vi "subVI_PhenotypeParalysis.vi"(6 "Start frame #":i32=50, 8 "Nb of frame to analyze":i32=580, 9 "Threshold Phenotype WT vs Paralyzed":dbl=120000.0 format="%#_13g", 10 "Threshold to binarize worm":i32, 11 "Path":path=path "C:/Users/aguillaume3/Desktop/TEST/Videos/20190614GA Serotonin paralysis on chip/N2/21 38 15 1 .avi") -> (2 "Mutant?":i32, 3 "Sum of diff":i32)   [LabVIEW 2019]
uses:
  <vilib>/vision/NI_Vision_Development_Module.lvlib
panel:
  out "Result":string
  out "Histogram":T1(graph)
  out "Image 4":T2(plugin-control)
  out "Frame #":i32
  out "Nb of frames":i32
  out "Image 3":T2(plugin-control)
  out "Image 2":T2(plugin-control)
  # "Inputs"
  # "Outputs"
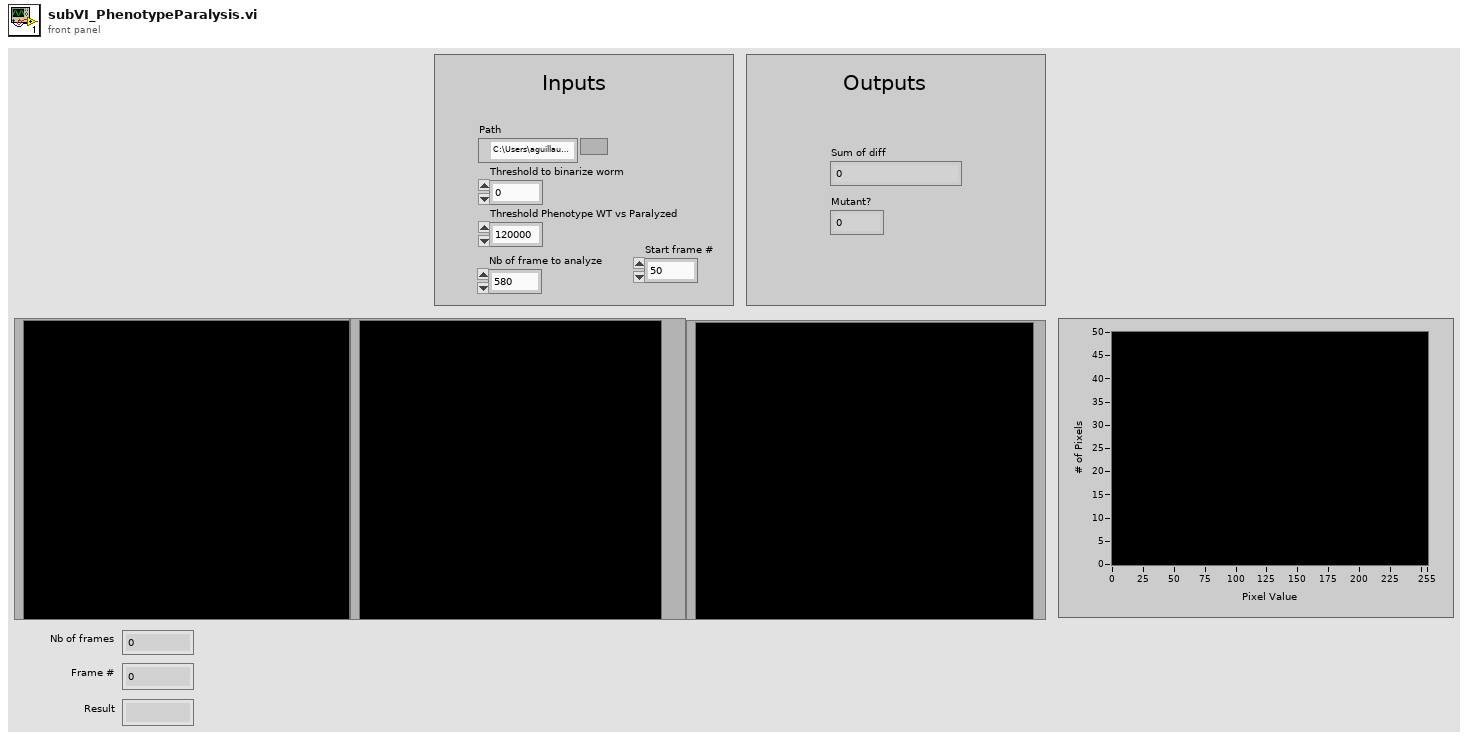
[diagram p1: front panel]
types:
  T1 = cluster{"Starting Value":sgl, "Incremental Value":sgl, "Histogram":u32[]}
  T2 = typedef "IMAQ Image.ctl" = refnum<image>
  T3 = typedef "Image Type" = u32
  T4 = typedef "IMAQ AVI2 Refnum.ctl" = refnum<k20>
  T5 = cluster{"Mean Value":sgl, "Standard Variation":sgl, "Minimal Value":sgl, "Maximal Value":sgl, "Area (calibrated)":sgl, "Area (pixels)":u32, "%":sgl, "Calibration Valid":bool}
  T6 = cluster{"histogram":u32[], "Minimal Value":sgl, "Maximal Value":sgl, "Starting Value":sgl, "Interval Width":sgl, "Mean Value":sgl, "Standard  Variation":sgl, "Area (pixels)":i32}
  T7 = cluster{"histogram[0]":u32, "histogram[1]":u32, "histogram[2]":u32, "histogram[3]":u32, "histogram[4]":u32, "histogram[5]":u32, "histogram[6]":u32, "histogram[7]":u32, "histogram[8]":u32}
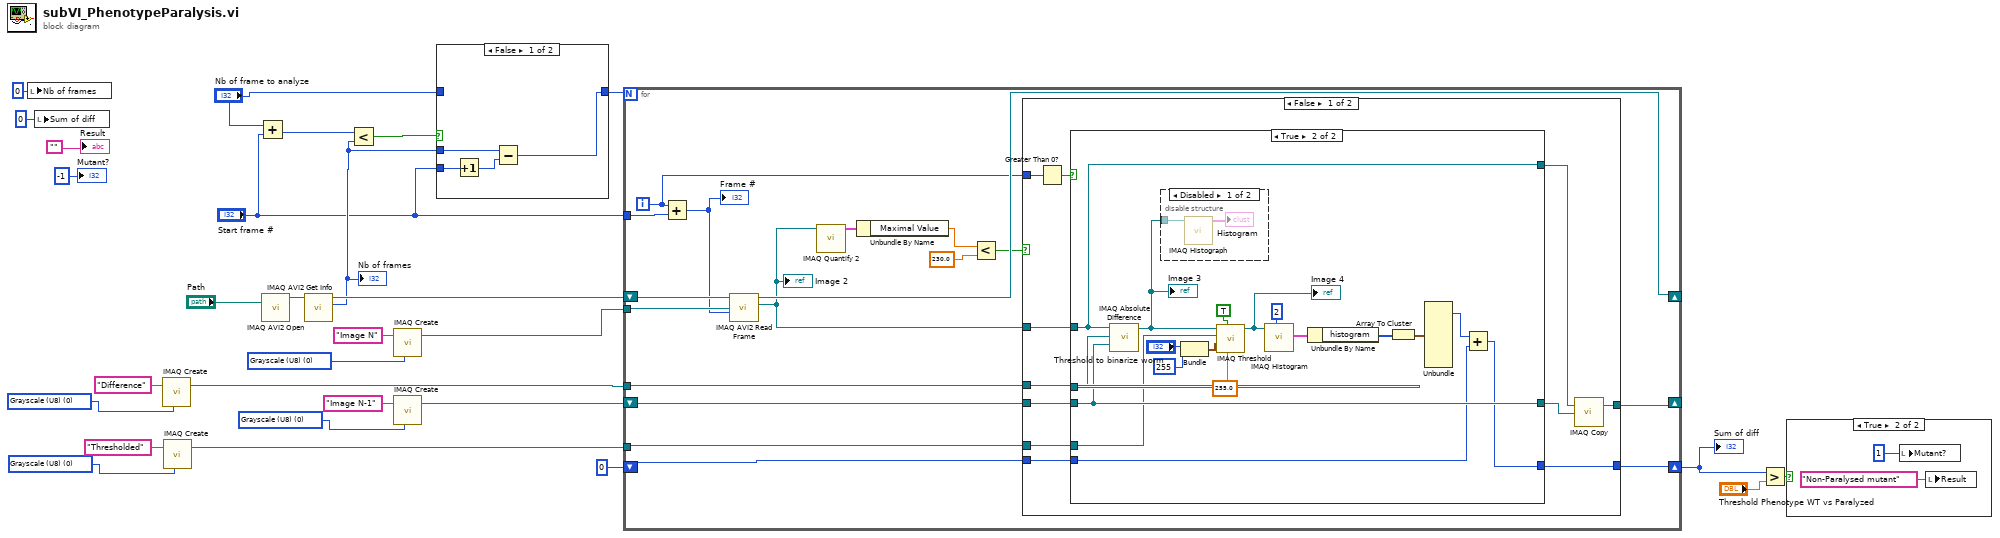
[diagram p0: block diagram]
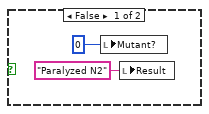
[diagram p3: hidden frame]
diagram:
  w18 = T3 0 items=["Grayscale (U8)", "Grayscale (I16)", "Grayscale (SGL)", "Complex (CSG)", "RGB (U32)", "HSL (U32)", "RGB (U64)", "Grayscale (U16)"] ("Image Type")
  w22 = T3 0 items=["Grayscale (U8)", "Grayscale (I16)", "Grayscale (SGL)", "Complex (CSG)", "RGB (U32)", "HSL (U32)", "RGB (U64)", "Grayscale (U16)"] ("Image Type")
  w25 = T3 0 items=["Grayscale (U8)", "Grayscale (I16)", "Grayscale (SGL)", "Complex (CSG)", "RGB (U32)", "HSL (U32)", "RGB (U64)", "Grayscale (U16)"] ("Image Type")
  w28 = T3 0 items=["Grayscale (U8)", "Grayscale (I16)", "Grayscale (SGL)", "Complex (CSG)", "RGB (U32)", "HSL (U32)", "RGB (U64)", "Grayscale (U16)"] ("Image Type")
  n1 = local write "Nb of frames"(0 ("Sum of diff")) -> ()
  n2 = local write "Sum of diff"(0 ("Sum of diff")) -> ()
  n3 = call "IMAQ Create"("Image Name"="Difference", "Image Type"=w22) -> ("New Image"=w21:T2)  [unwired: 3 in, 1 out]
  n4 = call "IMAQ Create"("Image Name"="Thresholded", "Image Type"=w18) -> ("New Image"=w17:T2)  [unwired: 3 in, 1 out]
  n5 = Add(x="Nb of frame to analyze", y="Start frame #") -> (x+y=w6:i32)
  n6 = call "IMAQ AVI2 Open"("AVI File Path"="Path") -> ("AVI Refnum"=w13:T4)  [unwired: 9 in, 1 out]
  n7 = call "IMAQ AVI2 Get Info"("AVI Refnum"=w13) -> ("Number of Frames"=w2:u32, "AVI Refnum (duplicate)"=w12:T4)  [unwired: 6 in, 3 out]
  "Nb of frames" <- w2
  n8 = Less?(x=w6, y=w2) -> (x < y?=w5:bool)
  n9 = call "IMAQ Create"("Image Name"="Image N", "Image Type"=w28) -> ("New Image"=w27:T2)  [unwired: 3 in, 1 out]
  n10 = call "IMAQ Create"("Image Name"="Image N-1", "Image Type"=w25) -> ("New Image"=w24:T2)  [unwired: 3 in, 1 out]
  n11 = case shown="False" w5 {
    tunnel: "Nb of frame to analyze" -> [_ w34]
    tunnel: [w32 w34] -> w3
    tunnel: w2 -> [w33 _]
    tunnel: "Start frame #" -> [w31 _]
    frame False {
      n12 = Increment(x=w31) -> (x+1=w30:i32)
      n13 = Subtract(x=w33, y=w30) -> (x-y=w32:u32)
    }
    frame True {
    }
  }
  n14 = for {
    N: w3 -> [_]
    shift-right: [w51] -> _
    shift-left: w12 -> [w50]
    tunnel: w27 -> [w49]
    shift-right: [w47] -> _
    shift-left: w24 -> [w48]
    tunnel: w21 -> [w46]
    shift-right: [w44] -> w10
    shift-left: 0 ("Numeric") -> [w45]
    tunnel: w17 -> [w42]
    tunnel: "Start frame #" -> [w40]
    i -> [w41]
    n15 = Add(x=w41, y=w40) -> (x+y=w43:i32)
    "Frame #" <- w43
    n16 = call "IMAQ AVI2 Read Frame"("Frame Number"=w43, "Image"=w49, "AVI Refnum"=w50) -> ("Image Out"=w38:T2, "AVI Refnum (duplicate)"=w51:T4)  [unwired: 6 in, 1 out]
    "Image 2" <- w38
    n17 = call "IMAQ Quantify 2"("Image"=w38) -> ("Global Report"=w39:T5)  [unwired: 8 in, 2 out]
    n18 = Unbundle By Name(w39) -> ("Maximal Value"=w37:sgl)
    n19 = Less?(x=w37, y=sgl 230.0) -> (x < y?=w35:bool)
    n20 = case shown="False" w35 {
      tunnel: w48 -> [w62 w87]
      tunnel: [w61 w87] -> w47
      tunnel: w46 -> [w60 _]
      tunnel: w45 -> [w59 w86]
      tunnel: [w58 w86] -> w44
      tunnel: w42 -> [w57 _]
      tunnel: w38 -> [w53 _]
      tunnel: w41 -> [w52 _]
      frame False {
        n21 = Greater Than 0?(x=w52) -> (x > 0?=w54:bool)
        n22 = case shown="True" w54 {
          tunnel: w62 -> [w64 w81]
          tunnel: w53 -> [w65 w83]
          tunnel: [w65 w83] -> w56
          tunnel: [w64 w81] -> w55
          tunnel: w60 -> [_ w82]
          tunnel: w59 -> [w63 w79]
          tunnel: [w63 w78] -> w58
          tunnel: w57 -> [_ w77]
          frame False {
          }
          frame True {
            n23 = call "IMAQ Absolute Difference"("Image Src A"=w83, "Image Dst"=w82, "Image Src B"=w81) -> ("Image Dst Out"=w69:T2)  [unwired: 4 in, 1 out]
            "Image 3" <- w69
            n24 = disable-structure shown="Disabled" {
              disable-tunnel: w69 -> [w85 _]
              frame Disabled {
                n25 = call "IMAQ Histograph"("Image"=w85) -> ("Histogram Graph"=→"Histogram":T1)  [unwired: 7 in, 3 out]
              }
              frame Enabled {
              }
            }
            n26 = Bundle("Threshold to binarize worm"="Threshold to binarize worm", 255) -> (w66:cluster{"Threshold to binarize worm":i32, i32})  [unwired: 1 in]
            n27 = call "IMAQ Threshold"("Replace Value"=sgl 255.0, "Keep/Replace Value (Replace)"=TRUE, "Range"=w66, "Image Dst"=w77, "Image Src"=w69) -> ("Image Dst Out"=w74:T2)  [unwired: 5 in, 1 out]
            "Image 4" <- w74
            n28 = call "IMAQ Histogram"("Number of Classes"=2, "Image"=w74) -> ("Histogram Report"=w80:T6)  [unwired: 8 in, 1 out]
            n29 = Unbundle By Name(w80) -> ("histogram"=w72:u32[])
            n30 = Array To Cluster(array=w72) -> (cluster=w71:T7)
            n31 = Unbundle(w71) -> ("histogram[1]"=w70:u32)  [unwired: 8 out]
            n32 = Add(x=w70, y=w79) -> (x+y=w78:u32)
          }
        }
        n33 = call "IMAQ Copy"("Image Dst"=w55, "Image Src"=w56) -> ("Image Dst Out"=w61:T2)  [unwired: 4 in, 1 out]
      }
      frame True {
      }
    }
  }
  "Sum of diff" <- w10
  n34 = Greater?(x=w10, y="Threshold Phenotype WT vs Paralyzed") -> (0:w7:bool)
  n35 = case shown="True" w7 {
    frame False {
      n36 = local write "Mutant?"(0 ("Sum of diff")) -> ()
      n37 = local write "Result"("Paralyzed N2" ("Result")) -> ()
    }
    frame True {
      n38 = local write "Mutant?"(1 ("Sum of diff")) -> ()
      n39 = local write "Result"("Non-Paralysed mutant" ("Result")) -> ()
    }
  }
  "Result" <- ""
  "Mutant?" <- -1 ("Result")
